vi "Get App Config.vi"(8 "error in (no error)":errorcluster) -> (0 "error out":errorcluster, 3 "Configuration":T1)   [LabVIEW 2018]
uses:
  Controls/App Configuration.ctl
  <vilib>/Utility/xml.llb/Read From XML File(string).vi
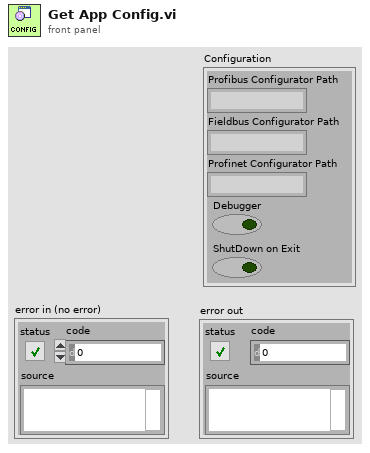
[diagram p1: front panel]
types:
  T1 = typedef "App Configuration.ctl" = cluster{"Profibus Configurator Path":string, "Fieldbus Configurator Path":string, "Profinet Configurator Path":string, "Debugger":bool, "ShutDown on Exit":bool}
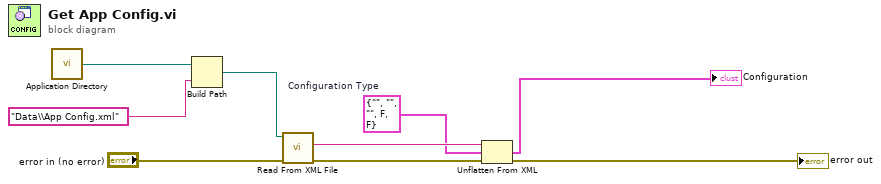
[diagram p0: block diagram]
diagram:
  w4 = T1 {"Profibus Configurator Path"="", "Fieldbus Configurator Path"="", "Profinet Configurator Path"="", "Debugger"=FALSE, "ShutDown on Exit"=FALSE}  # Configuration Type
  n1 = call <vilib>:"Application Directory.vi"() -> ("Application Directory"=w7:path)
  n2 = Build Path(base path=w7, name or relative path="Data\\App Config.xml") -> (appended path=w6:path)
  n3 = call-poly <vilib>:"Read From XML File.vi"("error in (no error)"="error in (no error)", "XML File Path"=w6) -> ("error out"=w3:errorcluster, "XML Elements"=w5:string)  [unwired: 7 in, 1 out]
  n4 = Unflatten From XML(xml string=w5, type=w4, error in (no error)=w3) -> (value=→"Configuration":T1, error out=→"error out":errorcluster)
